vi "LinearDiscriminantAnalysis.vi"(8 "error in":errorcluster) -> (0 "error out":errorcluster, 3 "out":refnum<class "LinearDiscriminantAnalysis.lvclass">)   [LabVIEW 2020]
doc: "Linear Discriminant Analysis\n\n A classifier with a linear decision boundary, generated by fitting class\n conditional densities to the data and using Bayes' rule.\n\n The model fits a Gaussian density to each class, assuming that all classes\n share the same covariance matrix.\n\n The fitted model can also be used to reduce the dimensionality of the input\n by projecting it to the most discriminative directions, using the\n `transform` method.\n\n .. versionadded:: 0.17\n *LinearDiscriminantAnalysis*.\n\n Read more in the :ref:`User Guide <lda_qda>`.\n\n Parameters\n ----------\n solver : {'svd', 'lsqr', 'eigen'}, default='svd'\n Solver to use, possible values:\n - 'svd': Singular value decomposition (default).\n Does not compute the covariance matrix, therefore this solver is\n recommended for data with a large number of features.\n - 'lsqr': Least squares solution.\n Can be combined with shrinkage or custom covariance estimator.\n - 'eigen': Eigenvalue decomposition.\n Can be combined with shrinkage or custom covariance estimator.\n\n shrinkage : 'auto' or float, default=None\n Shrinkage parameter, possible values:\n - None: no shrinkage (default).\n - 'auto': automatic shrinkage using the Ledoit-Wolf lemma.\n - float between 0 and 1: fixed shrinkage parameter.\n\n This should be left to None if `covariance_estimator` is used.\n Note that shrinkage works only with 'lsqr' and 'eigen' solvers.\n\n priors : array-like of shape (n_classes,), default=None\n The class prior probabilities. By default, the class proportions are\n inferred from the training data.\n\n n_components : int, default=None\n Number of components (<= min(n_classes - 1, n_features)) for\n dimensionality reduction. If None, will be set to\n min(n_classes - 1, n_features). This parameter only affects the\n `transform` method.\n\n store_covariance : bool, default=False\n If True, explicitely compute the weighted within-class covariance\n matrix when solver is 'svd'. The matrix is always computed\n and stored for the other solvers.\n\n .. versionadded:: 0.17\n\n tol : float, default=1.0e-4\n Absolute threshold for a singular value of X to be considered\n significant, used to estimate the rank of X. Dimensions whose\n singular values are non-significant are discarded. Only used if\n solver is 'svd'.\n\n .. versionadded:: 0.17\n\n covariance_estimator : covariance estimator, default=None\n If not None, `covariance_estimator` is used to estimate\n the covariance matrices instead of relying on the empirical\n covariance estimator (with potential shrinkage).\n The object should have a fit method and a ``covariance_`` attribute\n like the estimators in :mod:`sklearn.covariance`.\n if None the shrinkage parameter drives the estimate.\n\n This should be left to None if `shrinkage` is used.\n Note that `covariance_estimator` works only with 'lsqr' and 'eigen'\n solvers.\n\n .. versionadded:: 0.24\n\n Attributes\n ----------\n coef_ : ndarray of shape (n_features,) or (n_classes, n_features)\n Weight vector(s).\n\n intercept_ : ndarray of shape (n_classes,)\n Intercept term.\n\n covariance_ : array-like of shape (n_features, n_features)\n Weighted within-class covariance matrix. It corresponds to\n `sum_k prior_k * C_k` where `C_k` is the covariance matrix of the\n samples in class `k`. The `C_k` are estimated using the (potentially\n shrunk) biased estimator of covariance. If solver is 'svd', only\n exists when `store_covariance` is True.\n\n explained_variance_ratio_ : ndarray of shape (n_components,)\n Percentage of variance explained by each of the selected components.\n If ``n_components`` is not set then all components are stored and the\n sum of explained variances is equal to 1.0. Only available when eigen\n or svd solver is used.\n\n means_ : array-like of shape (n_classes, n_features)\n Class-wise means.\n\n priors_ : array-like of shape (n_classes,)\n Class priors (sum to 1).\n\n scalings_ : array-like of shape (rank, n_classes - 1)\n Scaling of the features in the space spanned by the class centroids.\n Only available for 'svd' and 'eigen' solvers.\n\n xbar_ : array-like of shape (n_features,)\n Overall mean. Only present if solver is 'svd'.\n\n classes_ : array-like of shape (n_classes,)\n Unique class labels.\n\n See Also\n --------\n QuadraticDiscriminantAnalysis : Quadratic Discriminant Analysis.\n\n \nAvailable methods:\nDecision Function\nFit\nPredict\nPredict Log Proba\nPredict Proba\nScore\nGet Attributes\nGet Params\nSet Params"
uses:
  LinearDiscriminantAnalysis.lvclass
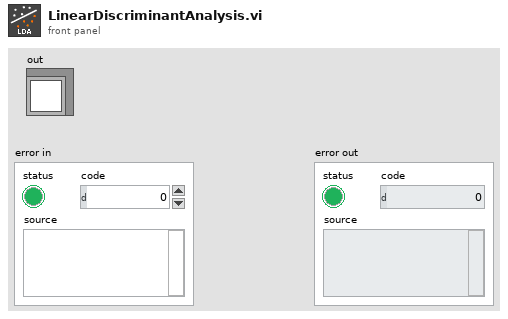
[diagram p1: front panel]
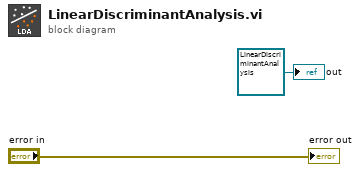
[diagram p0: block diagram]
diagram:
  "out" <- refnum<class "LinearDiscriminantAnalysis.lvclass"> refnum ("model")
  "error out" <- "error in"
